vi "NC_finddim.vi"(3 "name":string, 5 "NC_dimarray":cluster{"name":string, "size":u64}[](array[cluster])) -> (0 "dimid":i32, 1 "NC_dim":cluster{"name":string, "size":u64}, 2 "NC_dimarray out":cluster{"name":string, "size":u64}[](array[cluster]))   [LabVIEW 2016]
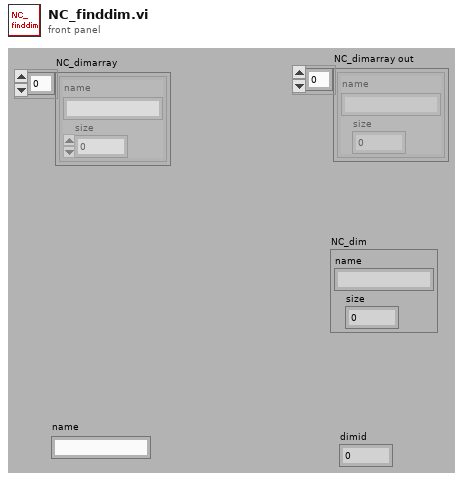
[diagram p1: front panel]
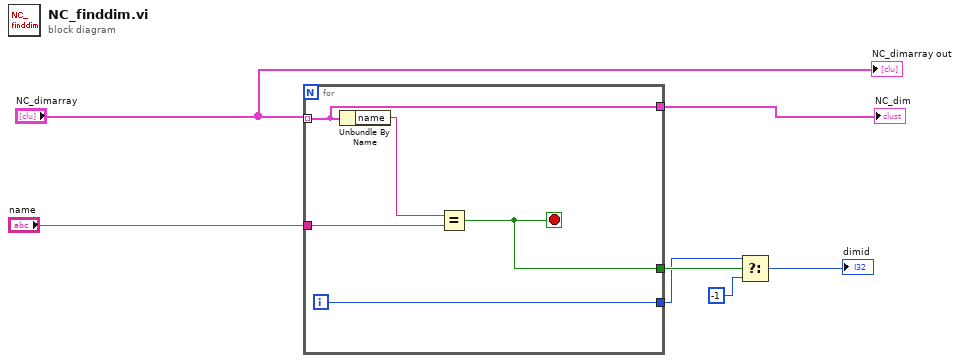
[diagram p0: block diagram]
diagram:
  n1 = for {
    tunnel: "NC_dimarray" -> [w8] mode=indexing
    tunnel: "name" -> [w11]
    tunnel: [w10] -> w3
    tunnel: [w9] -> w6
    tunnel: [w8] -> w1
    i -> [w10]
    stop <- w9 stop-if-true
    n2 = Unbundle By Name(w8) -> ("name"=w12:string)
    n3 = Equal?(x=w12, y=w11) -> (x = y?=w9:bool)
  }
  "NC_dim" <- w1
  n4 = Select(t=w3, s=w6, f=-1) -> (s? t:f=→"dimid":i32)
  "NC_dimarray out" <- "NC_dimarray"
